vi "DHE_reset_pci.vi"(0 "fd":i32, 7 "arguments":string, 11 "error in (no error)":errorcluster) -> (4 "fd out":i32, 8 "return value":i32, 15 "error out":errorcluster)   [LabVIEW 2016]
doc: "This VI closes the I/O interface with the instrument."
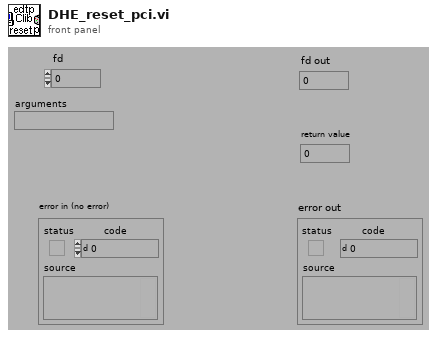
[diagram p1: front panel]
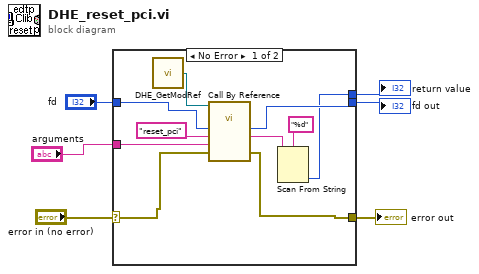
[diagram p0: block diagram]
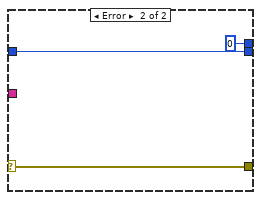
[diagram p2: hidden frame]
diagram:
  n1 = case shown="No Error" "error in (no error)" {
    selector: "error in (no error)" -> [w12 w17]
    tunnel: "fd" -> [w11 w19]
    tunnel: [w9 0] -> w5
    tunnel: [w8 w17] -> w4
    tunnel: [w10 w19] -> w3
    tunnel: "arguments" -> [w7 _]
    frame No Error {
      n2 = call "DHE_GetModRef.vi"() -> ("DHE_ModRef"=w16:refnum<vi>)  [unwired: 9 out]
      n3 = call-by-ref "?"(reference=w16, "error in (no error)"=w12, "arguments"=w7, "function"="reset_pci", "fd in"=w11) -> ("error out"=w8:errorcluster, "str result"=w14:string, "fd out"=w10:i32)  [unwired: 5 in, 3 out]
      n4 = Scan From String(format string="%d", input string=w14) -> (output 1=w9:i32)  [unwired: 2 in, 4 out]
    }
    frame Error {
    }
  }
  "error out" <- w4
  "return value" <- w5
  "fd out" <- w3
